vi "Check_meta_values.vi"(4 "Z-Position":dbl, 6 "Y-Position":dbl, 8 "X-Position":dbl, 9 "Z-Position_M":dbl, 10 "Y-Position_M":dbl, 11 "X-Position_M":dbl) -> (3 "Cancelled?":bool)   [LabVIEW 2011]
doc: "Let the user see the values of the meta data versus the currently entered values before choosing to load them."
panel:
  out "Z-Position D":dbl
  out "Y-Position D":dbl
  out "X-Position D":dbl
  in  "Cancel":bool
  in  "OK":bool
  # "Double Check your Meta Data Values\nwith the previously entered values.\nClick OK to accept Meta Values\nClick Cancel to keep old values."
  # "Difference"
  # "Original Value"
  # "MetaFile"
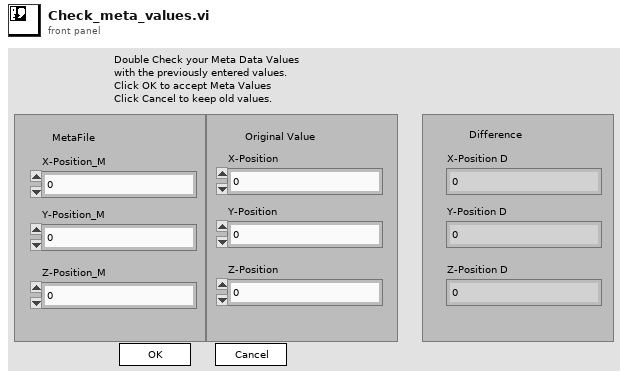
[diagram p1: front panel]
types:
  T1 = cluster{"X-Position":dbl, "Y-Position":dbl, "Z-Position":dbl}
  T2 = cluster{"X-Position_M":dbl, "Y-Position_M":dbl, "Z-Position_M":dbl}
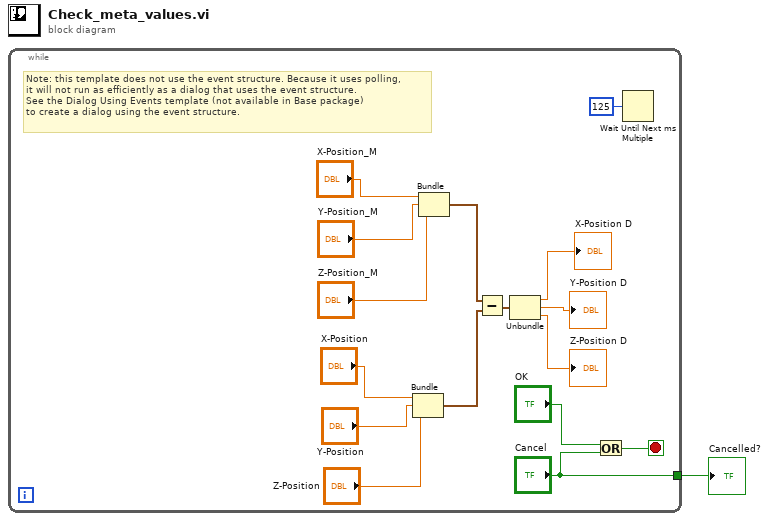
[diagram p0: block diagram]
diagram:
  n1 = while {
    tunnel: ["Cancel"] -> w1
    stop <- w16 stop-if-true
    # "Note: this template does not use the event structure. Because it uses polling, \nit will not run as efficiently as a dialog that uses the event structure.\nSee the Dialog Using Events template (not available in Base package) \nto create a dialog using the event structure."
    n2 = Bundle("X-Position"="X-Position", "Y-Position"="Y-Position", "Z-Position"="Z-Position") -> (w6:T1)  [unwired: 1 in]
    n3 = Bundle("X-Position_M"="X-Position_M", "Y-Position_M"="Y-Position_M", "Z-Position_M"="Z-Position_M") -> (w7:T2)  [unwired: 1 in]
    n4 = Subtract(x=w7, y=w6) -> (x-y=w5:cluster{dbl, dbl, dbl})
    n5 = Unbundle(w5) -> (→"X-Position D":dbl, →"Y-Position D":dbl, →"Z-Position D":dbl)
    n6 = Or(x="OK", y="Cancel") -> (x .or. y?=w16:bool)
    n7 = Wait Until Next ms Multiple(millisecond multiple=u32 125) -> ()  [unwired: 1 out]
  }
  "Cancelled?" <- w1
